vi "Instr_InitObject.vi"(8 "error in (no error)":errorcluster, 9 "Instrument Configuration":variant, 10 "Instrument address":refnum<visa-resource-name>, 11 "WK6425 in":refnum<class "WK6425.lvclass">) -> (0 "error out":errorcluster, 3 "WK6425 out":refnum<class "WK6425.lvclass">)   [LabVIEW 2013, in "WK6425.lvclass"]
uses:
  WK6425.lvclass
  LCRControl.lvclass
  InstrumentSetup.vi
  WK6425_CommandsGlobal.vi
  InstrControl.lvclass
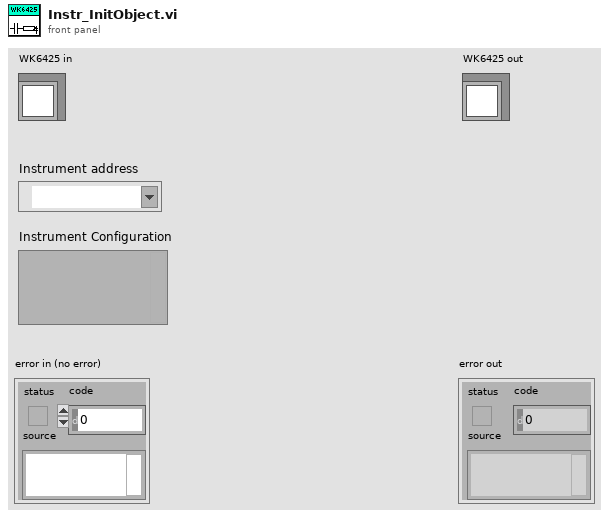
[diagram p1: front panel]
types:
  T1 = cluster{"RC Configuration":u16, "AC amplitude [V]":dbl, "AC frequency [Hz]":i32, "WK6425":refnum<class "WK6425.lvclass">}
  T2 = cluster{"Instrument name":string, "Command \"Initialise LCR\"":string, "Command \"OC Trim\"":string, "Command \"LCR Readout\"":string}
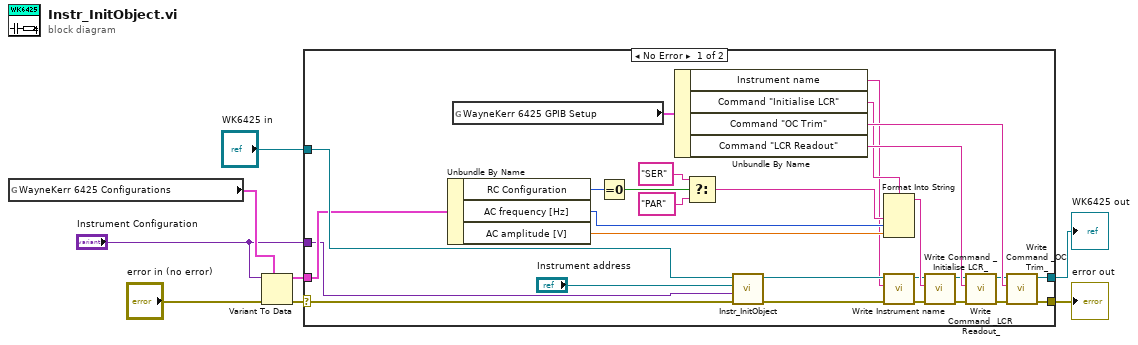
[diagram p0: block diagram]
diagram:
  n1 = global read "InstrumentSetup.vi" "WayneKerr 6425 Configurations"() -> (w5:T1)
  n2 = Variant To Data(error in="error in (no error)", type=w5, Variant="Instrument Configuration") -> (data=w4:T1, error out=w1:errorcluster)
  n3 = case shown="No Error" w1 {
    selector: w1 -> [w18 w38]
    tunnel: [w31 w38] -> w8
    tunnel: [w32 w37] -> w6
    tunnel: "WK6425 in" -> [w16 w37]
    tunnel: w4 -> [w10 _]
    tunnel: "Instrument Configuration" -> [w9 _]
    frame No Error {
      n4 = Unbundle By Name(w10) -> ("RC Configuration"=w28:u16, "AC frequency [Hz]"=w23:i32, "AC amplitude [V]"=w22:dbl)
      n5 = global read "WK6425_CommandsGlobal.vi" "WayneKerr 6425 GPIB Setup"() -> (w19:T2)
      n6 = Equal To 0?(x=w28) -> (x = 0?=w27:bool)
      n7 = Unbundle By Name(w19) -> ("Instrument name"=w14:string, "Command \"Initialise LCR\""=w21:string, "Command \"OC Trim\""=w35:string, "Command \"LCR Readout\""=w36:string)
      n8 = Select(t="SER", s=w27, f="PAR") -> (s? t:f=w24:string)
      n9 = call-parent "Instr_InitObject.vi"("error in (no error)"=w18, "Instrument Configuration"=w9, "Instrument address"="Instrument address", "LCRControl in"=w16) -> ("error out"=w13:errorcluster, "LCRControl out"=w15:refnum<class "WK6425.lvclass">)  [unwired: 6 in]
      n10 = Format Into String(format string=w21, w24, w23, w22) -> (resulting string=w20:string)  [unwired: 2 in, 1 out]
      n11 = call-dynamic "Write Instrument name.vi"("error in (no error)"=w13, "Instrument name"=w14, "InstControl in"=w15) -> ("error out"=w12:errorcluster, "InstControl out"=w11:refnum<class "WK6425.lvclass">)  [unwired: 7 in]
      n12 = call-dynamic "Write Command _Initialise LCR_.vi"("error in (no error)"=w12, "Command \"Initialise LCR\""=w20, "LCRControl in"=w11) -> ("error out"=w30:errorcluster, "LCRControl out"=w34:refnum<class "WK6425.lvclass">)  [unwired: 7 in]
      n13 = call-dynamic "Write Command _LCR Readout_.vi"("error in (no error)"=w30, "Command \"LCR Readout\""=w36, "LCRControl in"=w34) -> ("error out"=w29:errorcluster, "LCRControl out"=w33:refnum<class "WK6425.lvclass">)  [unwired: 7 in]
      n14 = call-dynamic "Write Command _OC Trim_.vi"("error in (no error)"=w29, "Command \"OC Trim\""=w35, "LCRControl in"=w33) -> ("error out"=w31:errorcluster, "LCRControl out"=w32:refnum<class "WK6425.lvclass">)  [unwired: 7 in]
    }
    frame Error {
    }
  }
  "error out" <- w8
  "WK6425 out" <- w6
